vi "Get MCP Gain Range.vi"(8 "error in (no error)":errorcluster, 10 "iHigh":i32, 11 "iLow":i32) -> (0 "error out":errorcluster, 1 "function return":u32, 2 "iHigh out":i32, 3 "iLow out":i32)   [LabVIEW 2014, in "atmcd32d.lvlib"]
doc: "unsigned int WINAPI GetMCPGainRange(int * iLow, int * iHigh);"
uses:
  atmcd32d.lvlib
  atmcd32d.dll
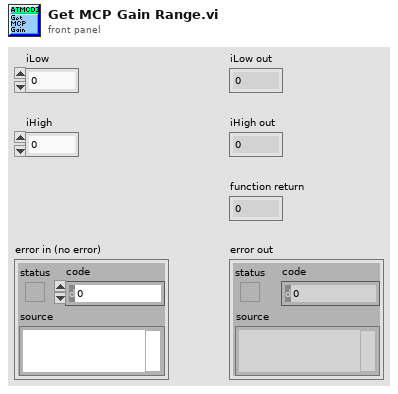
[diagram p1: front panel]
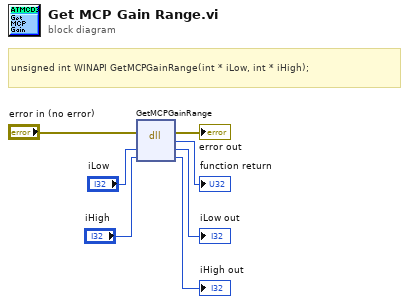
[diagram p0: block diagram]
diagram:
  # "unsigned int WINAPI GetMCPGainRange(int * iLow, int * iHigh);"
  n1 = dll-call lib="C:/Users/Bakir/Documents/Lambda2-Testing/lib/Andorlib/atmcd32d.*" fn="GetMCPGainRange"(error in="error in (no error)", "iLow"="iLow", "iHigh"="iHigh") -> (error out=→"error out":errorcluster, →"function return":u32, "iLow"=→"iLow out":i32, "iHigh"=→"iHigh out":i32)  [unwired: 2 in, 1 out]
